vi "Get Nsamples ILD420.vi"(0 "COM port":refnum<visa-resource-name>, 7 "N samples":i32=2000 min=0, 11 "Auto laser off":bool=TRUE) -> (4 "d (mm)":dbl[](array[numeric]), 15 "Error out":errorcluster)   [LabVIEW 2015]
panel:
  out "Samples acquired":i32
  out "Distance":dbl(graph)
  out "Bits":bool[][](array[boolean])
  # "mm"
  # "PN 12/08/2016"
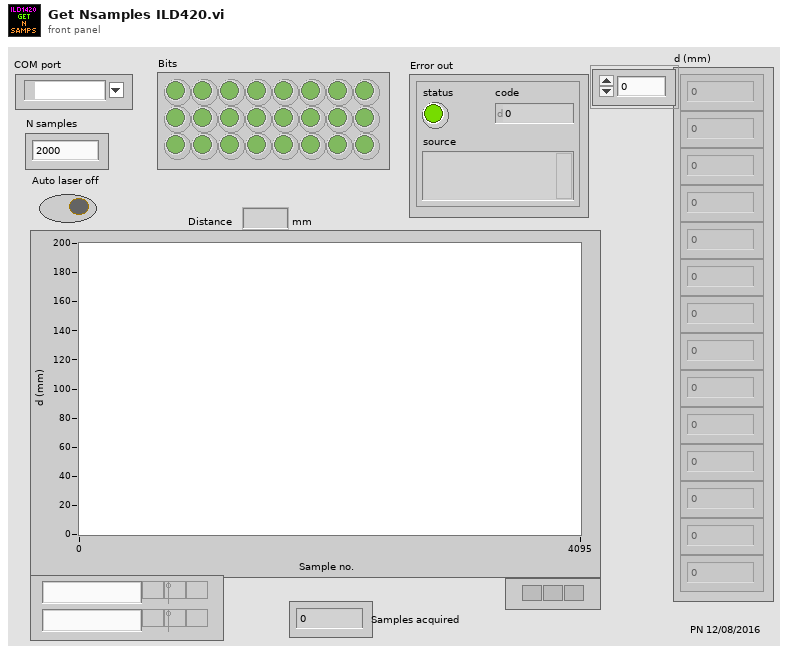
[diagram p1: front panel]
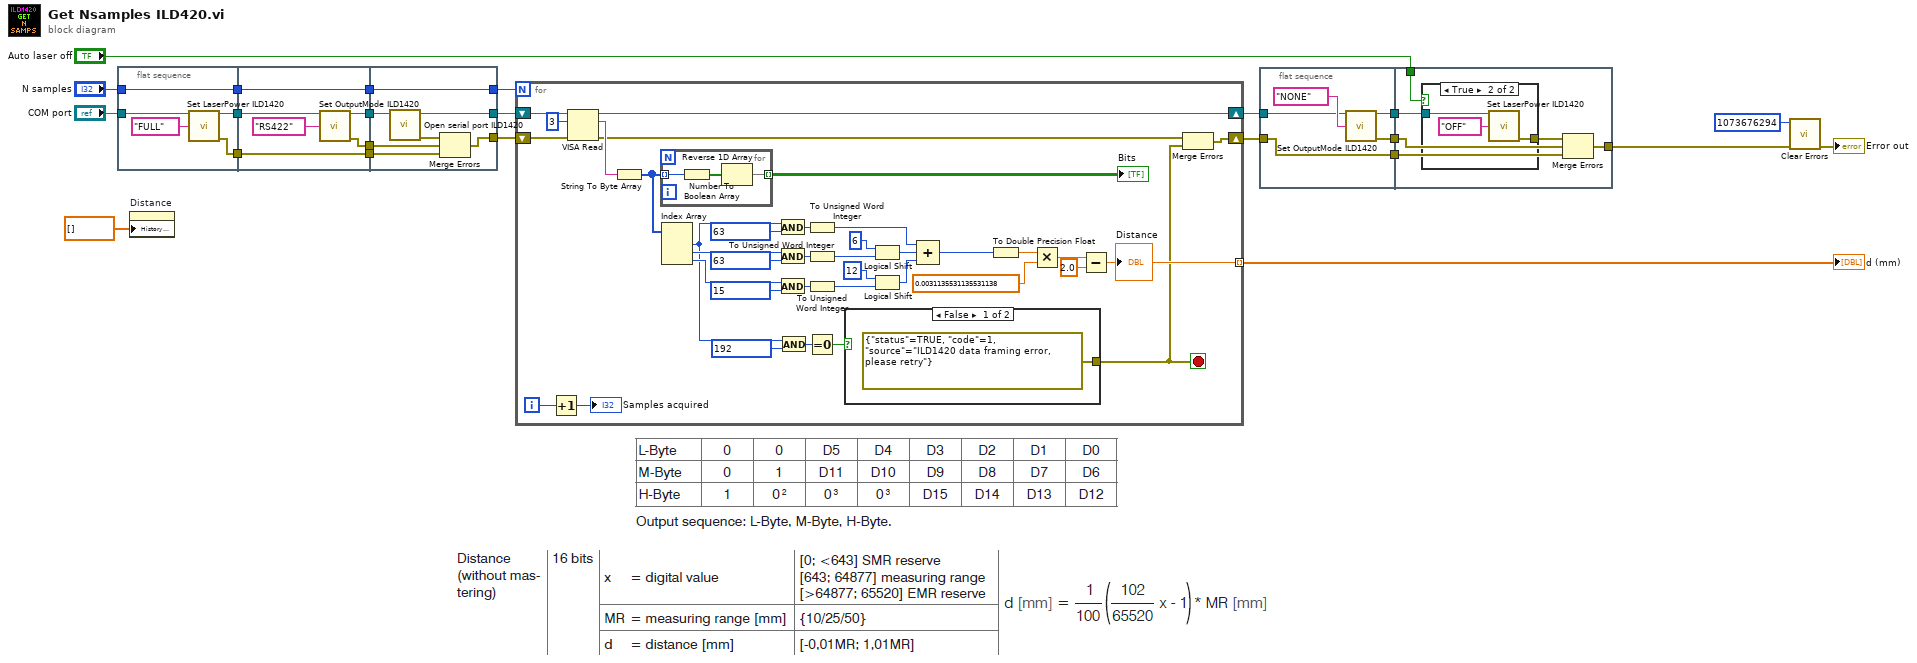
[diagram p0: block diagram]
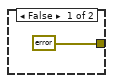
[diagram p2: hidden frame]
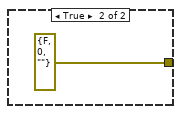
[diagram p3: hidden frame]
diagram:
  n1 = flat-sequence {
    tunnel: "N samples" -> [w27]
    tunnel: "COM port" -> [w26]
    tunnel: [w27] -> w9
    tunnel: [w26] -> w8
    tunnel: [w25] -> w6
    tunnel: [w31] -> w17
    tunnel: [w30] -> w16
    tunnel: [w29] -> w14
    tunnel: w9 -> [w29]
    tunnel: w8 -> [w31]
    tunnel: [w28] -> w7
    tunnel: w6 -> [w28]
    tunnel: [w39] -> w20
    tunnel: [w35] -> w18
    tunnel: w17 -> [w38]
    tunnel: w16 -> [w36]
    tunnel: w14 -> [w34]
    tunnel: [w34] -> w12
    tunnel: w7 -> [w33]
    frame #0 {
      n2 = call "Set LaserPower ILD1420.vi"("COM port"=w26, "Power"="FULL") -> ("Error out"=w25:errorcluster)  [unwired: 13 in]
    }
    frame #1 {
      n3 = call "Set OutputMode ILD1420.vi"("COM port"=w31, "Output mode"="RS422") -> ("Error out"=w30:errorcluster)  [unwired: 13 in]
    }
    frame #2 {
      n4 = call "Open serial port ILD1420.vi"("VISA resource name"=w38) -> ("Error out"=w37:errorcluster, "VISA resource name out"=w39:refnum<visa-resource-name>)  [unwired: 9 in]
      n5 = Merge Errors(w37, w36, w33) -> (w35:errorcluster)
    }
  }
  n6 = property on="Distance" class="WFChart (strict)"("History Data"=dbl[] []) -> ()  [unwired: 2 in, 2 out]
  n7 = for {
    N: w12 -> [_]
    shift-right: [w76] -> w21
    shift-left: w20 -> [w72]
    shift-right: [w43] -> w15
    shift-left: w18 -> [w71]
    tunnel: [w49] -> w23 mode=indexing
    i -> [w41]
    stop <- w42 stop-if-true
    n8 = Increment(x=w41) -> (x+1=→"Samples acquired":i32)
    n9 = VISA Read(VISA resource name=w72, byte count=u32 3, error in (no error)=w71) -> (VISA resource name out=w76:refnum<visa-resource-name>, read buffer=w73:string, error out=w44:errorcluster)  [unwired: 1 out]
    n10 = String To Byte Array(string=w73) -> (unsigned byte array=w50:u8[])
    n11 = for {
      tunnel: w50 -> [w81] mode=indexing
      tunnel: [w79] -> w74 mode=indexing
      n12 = Number To Boolean Array(number=w81) -> (Boolean array=w80:bool[])
      n13 = Reverse 1D Array(array=w80) -> (reversed array=w79:bool[])
    }
    "Bits" <- w74
    n14 = Index Array(array=w50) -> (element #1=w47:u8, element #2=w57:u8, element #3=w59:u8)  [unwired: 3 in]
    n15 = And(x=w47, y=u8 63) -> (x .and. y?=w67:u8)
    n16 = And(x=w57, y=u8 63) -> (x .and. y?=w60:u8)
    n17 = And(x=w59, y=u8 15) -> (x .and. y?=w63:u8)
    n18 = And(x=w47, y=u8 192) -> (x .and. y?=w46:u8)
    n19 = To Unsigned Word Integer(number=w67) -> (unsigned 16bit integer=w68:u16)
    n20 = To Unsigned Word Integer(number=w60) -> (unsigned 16bit integer=w69:u16)
    n21 = To Unsigned Word Integer(number=w63) -> (unsigned 16bit integer=w70:u16)
    n22 = Equal To 0?(x=w46) -> (x = 0?=w45:bool)
    n23 = case shown="False" w45 {
      tunnel: [errorcluster {"status"=TRUE, "code"=1, "source"="ILD1420 data framing error, please retry"} ("error out") errorcluster {"status"=FALSE, "code"=0, "source"=""} ("error out")] -> w42
      frame False {
      }
      frame True {
      }
    }
    n24 = Logical Shift(y=i16 6, x=w69) -> (x << y=w66:u16)
    n25 = Logical Shift(y=i16 12, x=w70) -> (x << y=w65:u16)
    n26 = Compound Arithmetic op=ADD(w68, w66, w65) -> (w64:u16)
    n27 = To Double Precision Float(number=w64) -> (double precision float=w51:dbl)
    n28 = Multiply(x=w51, y=0.0031135531135531138) -> (x*y=w53:dbl)
    n29 = Subtract(x=w53, y=2.0) -> (x-y=w49:dbl)
    "Distance" <- w49
    n30 = Merge Errors(w44, w42) -> (w43:errorcluster)
  }
  "d (mm)" <- w23
  n31 = flat-sequence {
    tunnel: w21 -> [w84]
    tunnel: w15 -> [w82]
    tunnel: [w84] -> w5
    tunnel: [w83] -> w4
    tunnel: [w82] -> w3
    tunnel: w5 -> [w91]
    tunnel: w4 -> [w89]
    tunnel: w3 -> [w88]
    tunnel: [w87] -> w2
    tunnel: "Auto laser off" -> [w86]
    frame #0 {
      n32 = call "Set OutputMode ILD1420.vi"("COM port"=w84, "Output mode"="NONE") -> ("Error out"=w83:errorcluster)  [unwired: 13 in]
    }
    frame #1 {
      n33 = case shown="True" w86 {
        tunnel: w91 -> [_ w94]
        tunnel: [errorcluster {"status"=FALSE, "code"=0, "source"=""} ("Error out") w93] -> w90
        frame False {
        }
        frame True {
          n34 = call "Set LaserPower ILD1420.vi"("COM port"=w94, "Power"="OFF") -> ("Error out"=w93:errorcluster)  [unwired: 13 in]
        }
      }
      n35 = Merge Errors(w90, w89, w88) -> (w87:errorcluster)
    }
  }
  n36 = call <vilib>:"Clear Errors.vi"("error in (no error)"=w2, "specific error code to clear (0: all)"=1073676294) -> ("error out"=→"Error out":errorcluster)  [unwired: 4 in, 1 out]
